vi "RFH-save-water_calib.vi"(5 "Save Name":string, 7 "Save Path":path=path "C:/projects/VNA/src/LabVIEW/spike", 8 "error in (no error)":errorcluster, 9 "Water temp":dbl=25.0, 10 "Common Format":T1) -> (0 "error out":errorcluster)   [LabVIEW 2020, in "RFH-Reflection_File_Handler.lvlib"]
uses:
  RFH-Reflection_File_Handler.lvlib
  RFH-common_data_format.ctl
  <vilib>/Utility/file.llb/Write Delimited Spreadsheet (DBL).vi
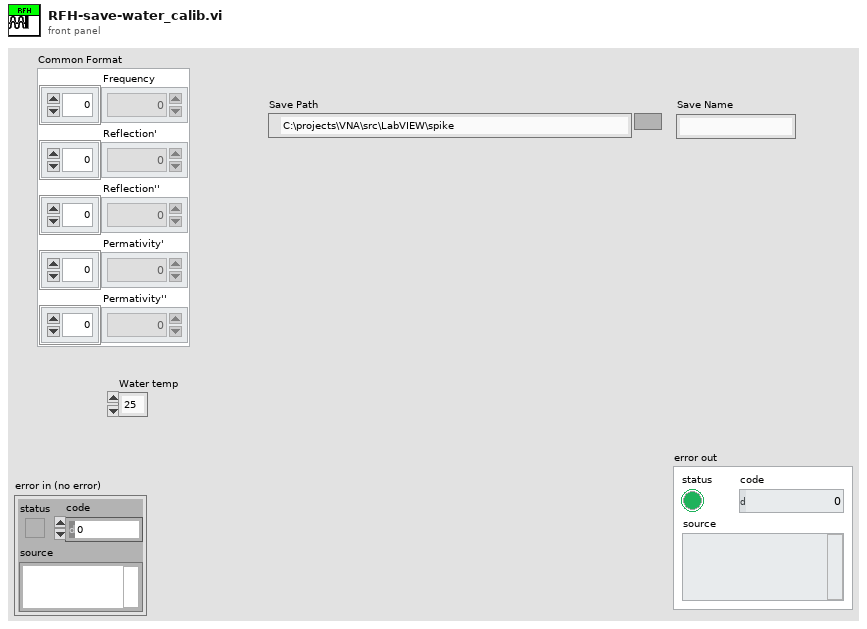
[diagram p1: front panel]
types:
  T1 = typedef "RFH-Reflection_File_Handler.lvlib/RFH-common_data_format.ctl" = cluster{"Frequency":dbl[], "Reflection'":dbl[], "Reflection''":dbl[], "Permativity'":dbl[], "Permativity''":dbl[]}
  T2 = enum16{"open", "replace", "create", "open or create", "replace or create", "replace or create with confirmation"}
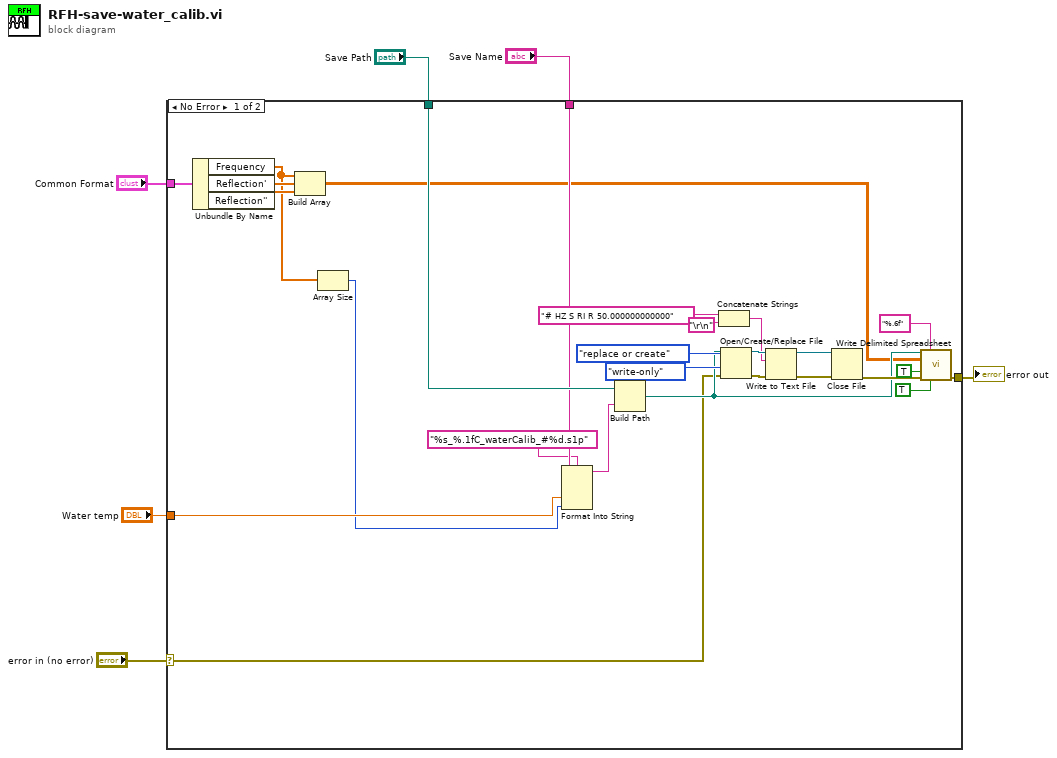
[diagram p0: block diagram]
diagram:
  n1 = case shown="No Error" "error in (no error)" {
    selector: "error in (no error)" -> [w14 w34]
    tunnel: "Save Path" -> [w33 _]
    tunnel: "Water temp" -> [w18 _]
    tunnel: "Save Name" -> [w17 _]
    tunnel: [w13 w34] -> w2
    tunnel: "Common Format" -> [w9 _]
    frame No Error {
      n2 = Unbundle By Name(w9) -> ("Frequency"=w8:dbl[], "Reflection'"=w12:dbl[], "Reflection''"=w11:dbl[])
      n3 = Build Array(w8, w12, w11) -> (w10:dbl[][])
      n4 = Array Size(array=w8) -> (size(s)=w7:i32)
      n5 = Format Into String(format string="%s_%.1fC_waterCalib_#%d.s1p", w17, w18, w7) -> (resulting string=w16:string)  [unwired: 2 in, 1 out]
      n6 = Build Path(base path=w33, name or relative path=w16) -> (appended path=w21:path)
      n7 = Concatenate Strings("# HZ S RI R 50.000000000000" ("text"), "\r\n") -> (w20:string)
      n8 = Open/Create/Replace File(file path (use dialog)=w21, error in=w14, operation (0:open)=T2."replace or create", access (0:read/write)=enum16{"read/write", "read-only", "write-only"}."write-only") -> (refnum out=w26:refnum<file>, error out=w25:errorcluster)  [unwired: 2 in, 1 out]
      n9 = Write to Text File(file (use dialog)=w26, text=w20, error in=w25) -> (refnum out=w28:refnum<file>, error out=w27:errorcluster)  [unwired: 1 in, 1 out]
      n10 = Close File(refnum=w28, error in=w27) -> (error out=w23:errorcluster)  [unwired: 1 out]
      n11 = call-poly <vilib>:"Write Delimited Spreadsheet.vi"("file path (dialog if empty)"=w21, "format (%.3f)"="%.6f", "2D data"=w10, "append to file? (new file:F)"=TRUE, "error in (no error)"=w23, "transpose? (no:F)"=TRUE) -> ("error out"=w13:errorcluster)  [unwired: 8 in, 1 out]
    }
    frame Error {
    }
  }
  "error out" <- w2
